vi "Radar_4channel_DAQ.vi"() -> ()   [LabVIEW 2017]
doc: "Personal Daq 54 example.\nTriggering is immediate and readings are returned 1 scan at a time as available.\nBe sure to use the Acquisition Stop control for proper shutdown."
uses:
  <vilib>/Utility/error.llb/DialogType.ctl
  <vilib>/DAQmx/read.llb/DAQmx Read (Analog 1D DBL NChan 1Samp).vi
  <vilib>/Analysis/2dsp.llb/Complex FFT.vi
  <vilib>/DAQmx/create/channels.llb/DAQmx Create Channel (AI-Voltage-Basic).vi
  <vilib>/DAQmx/configure/timing.llb/DAQmx Timing (Sample Clock).vi
  <vilib>/DAQmx/miscellaneous.llb/DAQmx Fill In Error Info.vi
  <vilib>/measure/madcrms.llb/Basic Averaged DC-RMS for 1 Chan.vi
  <vilib>/measure/NI_MAPro.lvlib
  <vilib>/Analysis/NI_AALPro.lvlib
panel:
  in  "Filename":path=path "C:/Users/rookie/Desktop/radar_data.lvm"
  in  "device":string(combo)="Dev1/ai0:7"
  in  "CH2 Q channel":i32=3
  in  "CH2 I channel":i32=2
  in  "CH1 Q channel":i32=1
  in  "CH1 I channel":i32
  in  "FFT length":i32=2048
  in  "buffer size":i32=256
  in  "samples per channel":i32=1
  in  "rate":dbl=20.0 format="%0.2f"
  in  "input terminal":T1(ring)=enum."RSE"
  in  "minimum value":dbl format="%0.2f"
  in  "maximum value":dbl=5.0 format="%0.2f"
  out "Spectrum 2":waveform(dbl)(graph)
  out "I/Q Signal 2":dynamicdata(graph)
  out "I/Q Signal 1":dynamicdata(graph)
  in  "Save Data":bool
  in  "stop":bool
  out "Spectrum 1":waveform(dbl)(graph)
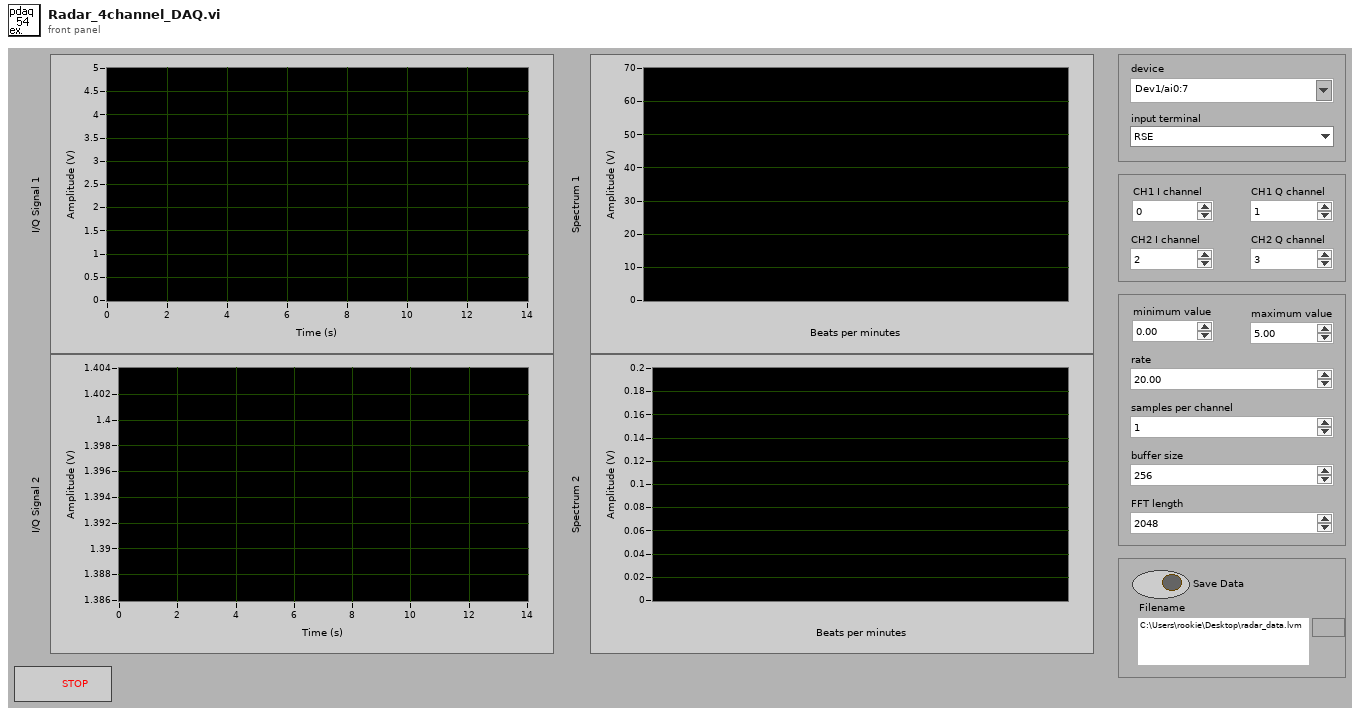
[diagram p1: front panel]
types:
  T1 = enum16{"Default", "RSE", "NRSE", "Differential", "Pseudodifferential"}
  T2 = typedef "DialogType.ctl" = u16
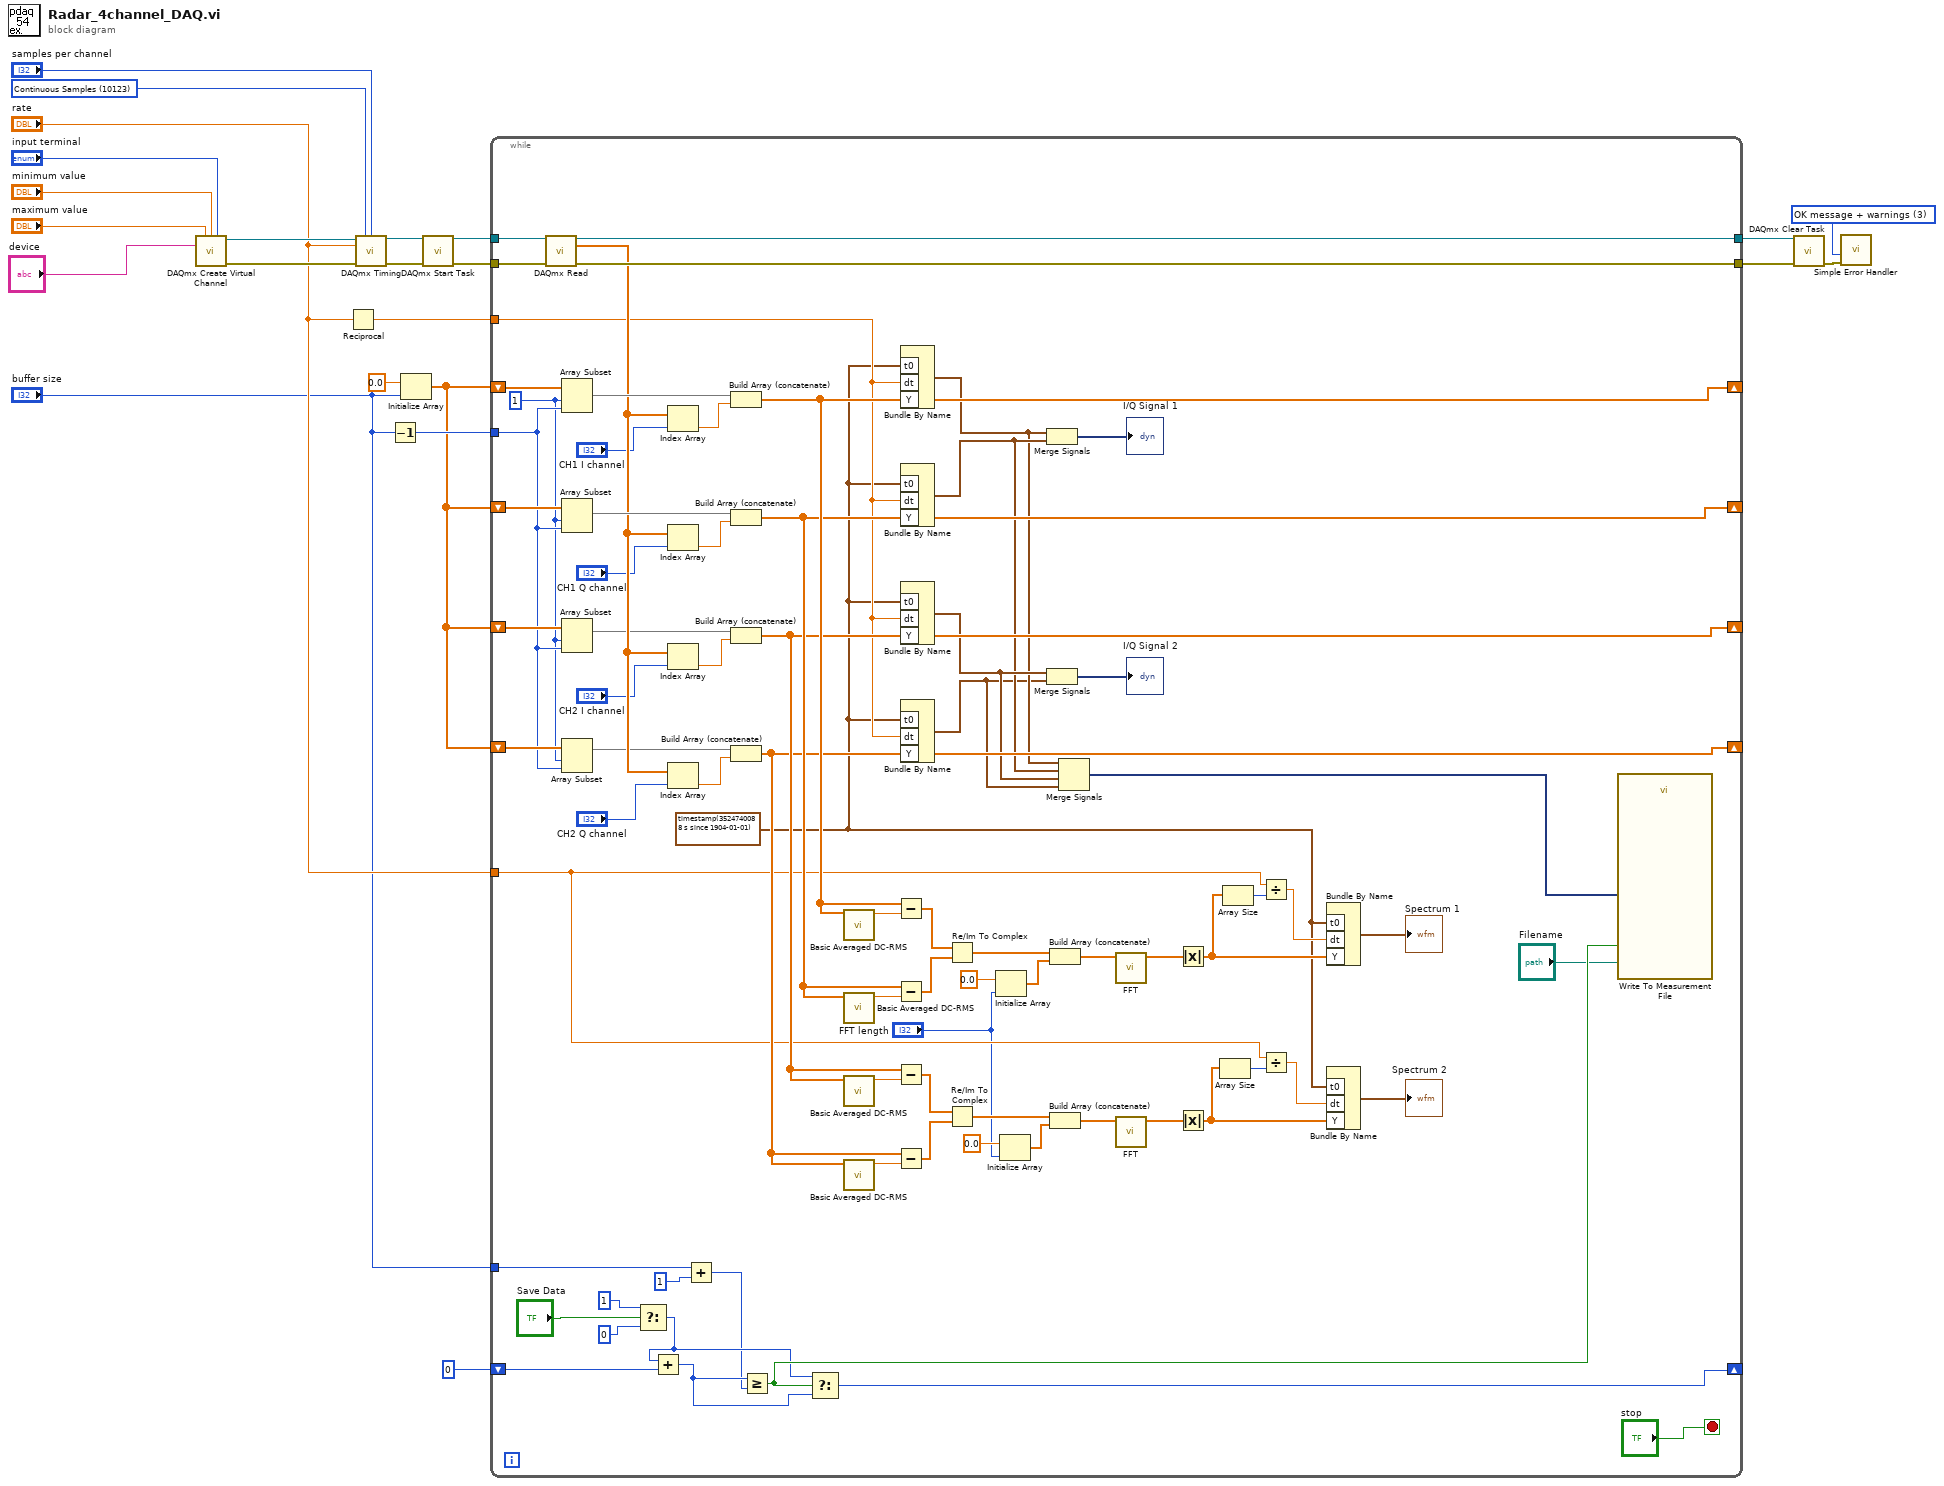
[diagram p0: block diagram]
diagram:
  w15 = T2 3 items=["no dialog", "OK message", "continue or stop message", "OK message + warnings", "continue/stop + warnings"] ("type of dialog (OK msg:1)")
  w8 = 10123 items=["Finite Samples"=10178, "Continuous Samples"=10123] ("sample mode")
  n1 = call-poly <vilib>:"DAQmx Create Virtual Channel.vi"("maximum value"="maximum value", "minimum value"="minimum value", "input terminal configuration"="input terminal", "physical channels"="device") -> ("task out"=w20:refnum<k21>, "error out"=w21:errorcluster)  [unwired: 5 in, 5 out]
  n2 = Reciprocal(x="rate") -> (1/x=w9:dbl)
  n3 = call-poly <vilib>:"DAQmx Timing.vi"("task/channels in"=w20, "sample mode"=w8, "samples per channel"="samples per channel", "rate"="rate", "error in"=w21) -> ("task out"=w19:refnum<k21>, "error out"=w18:errorcluster)  [unwired: 2 in, 7 out]
  n4 = Decrement(x="buffer size") -> (x-1=w22:i32)
  n5 = Initialize Array(0.0 ("element"), "buffer size") -> (w10:dbl[])
  n6 = call <vilib>:"DAQmx Start Task.vi"("task/channels in"=w19, "error in"=w18) -> ("task out"=w17:refnum<k21>, "error out"=w16:errorcluster)  [unwired: 12 out]
  n7 = while {
    shift-right: [w89] -> _
    shift-left: w10 -> [w100]
    tunnel: w22 -> [w67]
    shift-right: [w88] -> _
    shift-left: w10 -> [w98]
    tunnel: w17 -> [w87]
    tunnel: w16 -> [w86]
    tunnel: w9 -> [w35]
    tunnel: [w85] -> w14
    tunnel: [w84] -> w13
    tunnel: "buffer size" -> [w33]
    shift-right: [w76] -> _
    shift-left: 0 -> [w78]
    shift-right: [w60] -> _
    shift-left: w10 -> [w69]
    shift-right: [w59] -> _
    shift-left: w10 -> [w68]
    tunnel: "rate" -> [w31]
    stop <- "stop" stop-if-true
    w34 = timestamp(3524740088.296 s since 1904-01-01) ("t0")
    w30 = 1 ("index")
    n8 = call-poly <vilib>:"DAQmx Read.vi"("task/channels in"=w87, "error in"=w86) -> ("task out"=w85:refnum<k21>, "data"=w66:dbl[], "error out"=w84:errorcluster)  [unwired: 11 out]
    n9 = Array Subset(array=w100, index=w30, length=w67) -> (w99:dbl[])
    n10 = Array Subset(array=w98, index=w30, length=w67) -> (w97:dbl[])
    n11 = Array Subset(array=w69, index=w30, length=w67) -> (w36:dbl[])
    n12 = Array Subset(array=w68, index=w30, length=w67) -> (w65:dbl[])
    n13 = Select(t=1, s="Save Data", f=0) -> (s? t:f=w72:i32)
    n14 = Add(x=w72, y=w78) -> (x+y=w77:i32)
    n15 = Index Array(array=w66, index="CH1 I channel") -> (element=w40:dbl)
    n16 = Index Array(array=w66, index="CH1 Q channel") -> (element=w39:dbl)
    n17 = Index Array(array=w66, index="CH2 I channel") -> (element=w38:dbl)
    n18 = Index Array(array=w66, index="CH2 Q channel") -> (element=w37:dbl)
    n19 = Add(x=w33, y=1 ("index")) -> (x+y=w63:i32)
    n20 = Build Array (concatenate)(w99, w40) -> (w89:dbl[])
    n21 = Build Array (concatenate)(w97, w39) -> (w88:dbl[])
    n22 = Build Array (concatenate)(w36, w38) -> (w60:dbl[])
    n23 = Build Array (concatenate)(w65, w37) -> (w59:dbl[])
    n24 = Greater Or Equal?(x=w77, y=w63) -> (x >= y?=w75:bool)
    n25 = Select(t=w72, s=w75, f=w77) -> (s? t:f=w76:i32)
    n26 = call-poly <vilib>:"Basic Averaged DC-RMS.vi"("signal in"=w89) -> ("DC value"=w93:dbl)  [unwired: 4 in, 6 out]
    n27 = call-poly <vilib>:"Basic Averaged DC-RMS.vi"("signal in"=w88) -> ("DC value"=w94:dbl)  [unwired: 4 in, 6 out]
    n28 = call-poly <vilib>:"Basic Averaged DC-RMS.vi"("signal in"=w60) -> ("DC value"=w61:dbl)  [unwired: 4 in, 6 out]
    n29 = call-poly <vilib>:"Basic Averaged DC-RMS.vi"("signal in"=w59) -> ("DC value"=w62:dbl)  [unwired: 4 in, 6 out]
    n30 = Subtract(x=w89, y=w93) -> (x-y=w82:dbl[])
    n31 = Subtract(x=w88, y=w94) -> (x-y=w81:dbl[])
    n32 = Subtract(x=w60, y=w61) -> (x-y=w57:dbl[])
    n33 = Subtract(x=w59, y=w62) -> (x-y=w58:dbl[])
    n34 = Bundle By Name("t0"=w34, "dt"=w35, "Y"=w89) -> (w51:waveform(dbl))  [unwired: 1 out]
    n35 = Bundle By Name("t0"=w34, "dt"=w35, "Y"=w88) -> (w52:waveform(dbl))  [unwired: 1 out]
    n36 = Bundle By Name("t0"=w34, "dt"=w35, "Y"=w60) -> (w53:waveform(dbl))  [unwired: 1 out]
    n37 = Bundle By Name("t0"=w34, "dt"=w35, "Y"=w59) -> (w32:waveform(dbl))  [unwired: 1 out]
    n38 = Re/Im To Complex(1:w81, 2:w82) -> (0:w95:cdb[])
    n39 = Re/Im To Complex(1:w58, 2:w57) -> (0:w41:cdb[])
    n40 = Initialize Array(0.0 ("element"), "FFT length") -> (w56:dbl[])
    n41 = Initialize Array(0.0 ("element"), "FFT length") -> (w49:dbl[])
    n42 = Merge Signals(w51, w52) -> (→"I/Q Signal 1":dynamicdata)
    n43 = Merge Signals(w53, w32) -> (→"I/Q Signal 2":dynamicdata)
    n44 = Build Array (concatenate)(w95, w56) -> (w90:cdb[])
    n45 = Build Array (concatenate)(w41, w49) -> (w45:cdb[])
    n46 = Merge Signals(w51, w52, w53, w32) -> (w50:dynamicdata)
    n47 = call-poly <vilib>:"FFT.vi"("X"=w90) -> ("FFT {X}"=w92:cdb[])  [unwired: 2 in, 8 out]
    n48 = call-poly <vilib>:"FFT.vi"("X"=w45) -> ("FFT {X}"=w43:cdb[])  [unwired: 2 in, 8 out]
    n49 = Absolute Value(x=w92) -> (abs(x)=w70:dbl[])
    n50 = Absolute Value(x=w43) -> (abs(x)=w48:dbl[])
    n51 = Array Size(array=w48) -> (size(s)=w44:i32)
    n52 = Array Size(array=w70) -> (size(s)=w91:i32)
    n53 = Divide(x=w31, y=w91) -> (x/y=w79:dbl)
    n54 = Divide(x=w31, y=w44) -> (x/y=w47:dbl)
    n55 = Bundle By Name("t0"=w34, "dt"=w79, "Y"=w70) -> (→"Spectrum 1":waveform(dbl))  [unwired: 1 out]
    n56 = Bundle By Name("t0"=w34, "dt"=w47, "Y"=w48) -> (→"Spectrum 2":waveform(dbl))  [unwired: 1 out]
    n57 = call "Write To Measurement File"("Signals"=w50, "Enable"=w75, "Filename"="Filename") -> ()  [unwired: 14 in, 3 out]
  }
  n58 = call <vilib>:"DAQmx Clear Task.vi"("task in"=w14, "error in"=w13) -> ("error out"=w12:errorcluster)  [unwired: 13 out]
  n59 = call <vilib>:"Simple Error Handler.vi"("type of dialog (OK msg:1)"=w15, "error in (no error)"=w12) -> ()  [unwired: 8 out]
